vi "003 Bundle unbundle.vi"() -> ()   [LabVIEW 2019]
panel:
  out "cluster mod":T1
  out "Boolean 2":bool
  out "Numeric":dbl
  out "output cluster":cluster{"Boolean 1":bool, "Slide":dbl}
  in  "Cluster":T1 {"Slide" scale=0.0..10.0}
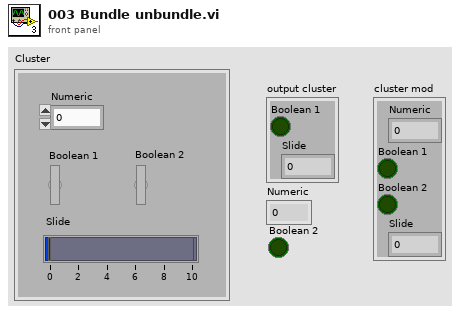
[diagram p1: front panel]
types:
  T1 = cluster{"Numeric":dbl, "Boolean 1":bool, "Boolean 2":bool, "Slide":dbl}
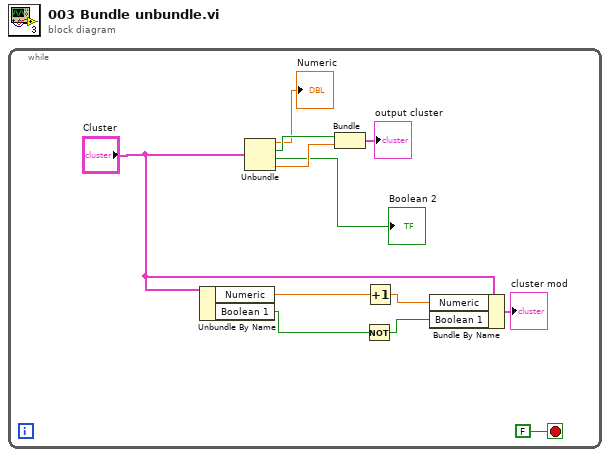
[diagram p0: block diagram]
diagram:
  n1 = while {
    stop <- FALSE stop-if-true
    n2 = Unbundle By Name("Cluster") -> ("Numeric"=w6:dbl, "Boolean 1"=w5:bool)
    n3 = Unbundle("Cluster") -> ("Numeric"=→"Numeric":dbl, "Boolean 1"=w12:bool, "Boolean 2"=→"Boolean 2":bool, "Slide"=w11:dbl)
    n4 = Bundle("Boolean 1"=w12, "Slide"=w11) -> (→"output cluster":cluster{"Boolean 1":bool, "Slide":dbl})  [unwired: 1 in]
    n5 = Not(x=w5) -> (.not. x?=w2:bool)
    n6 = Increment(x=w6) -> (x+1=w3:dbl)
    n7 = Bundle By Name(cluster="Cluster", "Numeric"=w3, "Boolean 1"=w2) -> (→"cluster mod":T1)
  }
